vi "Graph - Silver Simple.vi"() -> ()   [LabVIEW 2011]
doc: "Sample numeric display item."
uses:
  Silver Support LLB.llb/cluster_Screen Item Settings.ctl
  Silver Support LLB.llb/cluster_Graph Scale Settings.ctl
  Silver Support LLB.llb/cluster_Graph Plot Settings.ctl
  Silver Support LLB.llb/cluster_Graph Handler Message.ctl
  Silver Support LLB.llb/enum_Graph Handler Message.ctl
  Silver Support LLB.llb/sub_Display Template Handler Graph.vi
  Silver Support LLB.llb/sub_Display Template Data Handler Graph.vi
panel:
  out "Graph":waveform(dbl)[](graph)
  out "Label":string="Numeric"
  out "Data Lost":bool
  out "Y.Autoscale":bool
  in  "Y.Scale.Once":bool
  in  "Y.Scale.Auto":bool
  out "X.Autoscale":bool
  in  "X.Scale.Once":bool
  in  "X.Scale.Auto":bool
  in  "Legend":bool
  in  "Setup":bool
  in  "Hold":bool
  in  "Item.Data":T1
  # "Autoscale X"
  # "Autoscale Y"
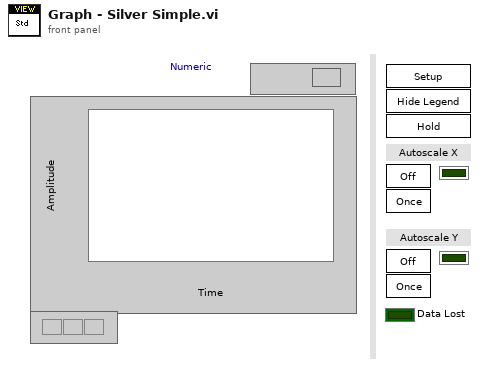
[diagram p1: front panel]
types:
  T1 = typedef "cluster_Screen Item Settings.ctl" = cluster{"Template VI":string, "Position X":i32, "Position Y":i32, "Custom":string, "Show Title Bar":bool, "ID":i32, "Always On Top":bool, "Allow Resize":bool, "Allow Minimize":bool, "Allow Close":bool, "Size to Screen":bool, "Screen.ID":i32, "State":enum16{"Normal", "New"}, "Title":string, "Window Bounds":cluster{"[0]":i16, "[1]":i16, "[2]":i16, "[3]":i16}, "Channel Ref":u64, "Unit":string, "Default Units?":bool, "Flash Limit?":bool, "Color 1":u32, "Color 2":u32, "Color 3":u32, "Color 4":u32, "Bck Color":u32, "Fore Color":u32, "Limit 1":dbl, "Limit 2":dbl, "Limit 3":dbl, "Limit 4":dbl, "Limit Mode 1":i32, "Limit Mode 2":i32, "Limit Mode 3":i32, "Limit Mode 4":i32, "Scale Precision":i32, "Scale Min":dbl, "Scale Max":dbl, "Format":i32, "Precision":i32, "Background Type":i32, "IDs":i32[], "Units":string[], "Labels":string[], "Scale Factor":dbl, "Scale Offset":dbl, "YScale Index":u32[], "XScale":T2, "YScales":T2[], "Plots":T3[], "Update Period":dbl, "History Length":dbl, "My.Ref":refnum<vi>, "Is Control?":bool, "Channel Paths":string[], "Custom Data":variant}
  T2 = typedef "cluster_Graph Scale Settings.ctl" = cluster{"Format":u8, "Precision":u8, "Fit":u8, "Label":string, "Use Default Label":bool, "Label Visible":bool, "Min":dbl, "Max":dbl}
  T3 = typedef "cluster_Graph Plot Settings.ctl" = cluster{"Bar Style":u8, "Fill To":i16, "Fill/PtColor":u32, "Line Style":u8, "Line Width":u8, "Color":u32, "Interp":u8, "Point Style":u8}
  T4 = typedef "cluster_Graph Handler Message.ctl" = cluster{"Message":T5, "Data":variant}
  T5 = typedef "enum_Graph Handler Message.ctl" = enum16{"None", "Stop", "Hold", "Update Channels", "New Settings", "Control Value", "Edit Value"}
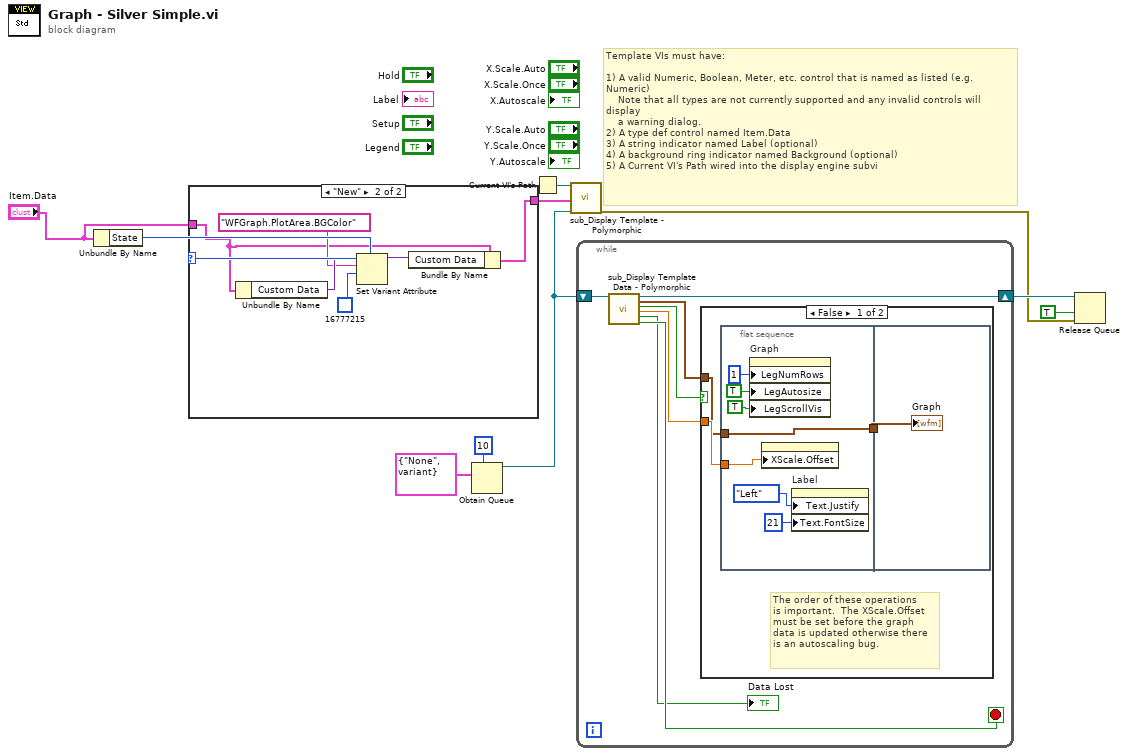
[diagram p0: block diagram]
diagram:
  # "Template VIs must have:\n\n1) A valid Numeric, Boolean, Meter, etc. control that is named as listed (e.g. Numeric)\n    Note that all types are not currently supported and any invalid controls will display\n    a warning dialog.\n2) A type def control named Item.Data\n3) A string indicator named Label (optional)\n4) A background ring indicator named Background (optional)\n5) A Current VI's Path wired into the display engine subvi"
  n1 = Unbundle By Name("Item.Data") -> ("State"=w3:enum16{"Normal", "New"})
  n2 = case shown="\"New\"" w3 {
    tunnel: "Item.Data" -> [w11 w13]
    tunnel: [w11 w12] -> w1
    frame "Normal", Default {
    }
    frame "New" {
      n3 = Unbundle By Name(w13) -> ("Custom Data"=w17:variant)
      n4 = Set Variant Attribute(Variant=w17, name="WFGraph.PlotArea.BGColor", value=u32 16777215) -> (Variant out=w14:variant)  [unwired: 1 in, 2 out]
      n5 = Bundle By Name(cluster=w13, "Custom Data"=w14) -> (w12:T1)
    }
  }
  n6 = Obtain Queue(max queue size (-1, unlimited)=10, element data type=T4 {"Message"=enum."None", "Data"=variant} ("Message")) -> (queue out=w5:refnum<queue>)  [unwired: 2 in, 3 out]
  n7 = Current VI's Path() -> (path=w10:path)
  n8 = call-poly "sub_Display Template - Polymorphic.vi"("Parent.Path"=w10, "Item.Data"=w1, "queue"=w5) -> ("error out"=w4:errorcluster)  [unwired: 16 out]
  n9 = while {
    shift-right: [w24] -> w9
    shift-left: w5 -> [w23]
    stop <- w19 stop-if-true
    n10 = call-poly "sub_Display Template Data - Polymorphic.vi"("queue"=w23) -> ("queue out"=w24:refnum<queue>, "Graph.Data"=w22:waveform(dbl)[], "Hold"=w20:bool, "XScale.Offset"=w21:dbl, "Data Lost"=→"Data Lost":bool, "Stop"=w19:bool)  [unwired: 13 out]
    n11 = case shown="False" w20 {
      tunnel: w21 -> [w27 _]
      tunnel: w22 -> [w26 _]
      frame False {
        # "The order of these operations\nis important.  The XScale.Offset\nmust be set before the graph\ndata is updated otherwise there\nis an autoscaling bug."
        n12 = flat-sequence {
          tunnel: w27 -> [w33]
          tunnel: w26 -> [w34]
          tunnel: [w34] -> w25
          tunnel: w25 -> [w35]
          frame #0 {
            n13 = property on="Graph" class="WFGraph (strict)"("LegNumRows"=u32 1 ("Legend:Number of Rows"), "LegAutosize"=TRUE ("Legend:Autosize"), "LegScrollVis"=TRUE ("Legend:Autosize")) -> ()  [unwired: 2 in, 2 out]
            n14 = property on="Graph" class="WFGraph (strict)"("XScale.Offset"=w33) -> ()  [unwired: 2 in, 2 out]
            n15 = property on="Label" class="Str"("Text.Justify"=enum16{"Left", "Center", "Right"}."Left" ("Text.Justification"), "Text.FontSize"=u32 21 ("Text.Font:Size")) -> ()  [unwired: 2 in, 2 out]
          }
          frame #1 {
            "Graph" <- w35
          }
        }
      }
      frame True {
      }
    }
  }
  n16 = Release Queue(queue=w9, force destroy? (F)=TRUE, error in (no error)=w4) -> ()  [unwired: 3 out]
